vi "Apply Gate.vi"(8 "nramp":i32, 9 "Waveform in":dbl[](array[numeric])) -> (1 "Gated waveform":dbl[](array[numeric]))   [LabVIEW 2020]
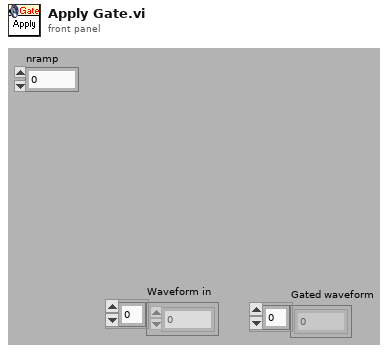
[diagram p1: front panel]
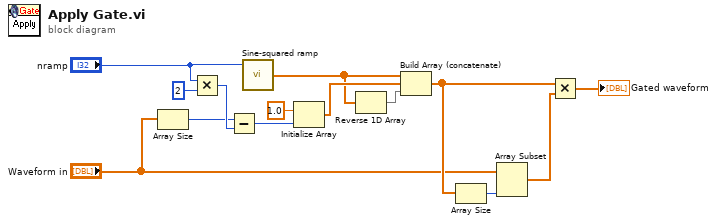
[diagram p0: block diagram]
diagram:
  n1 = Array Size(array="Waveform in") -> (size(s)=w2:i32)
  n2 = Multiply(x="nramp", y=2) -> (x*y=w13:i32)
  n3 = Subtract(x=w2, y=w13) -> (x-y=w12:i32)
  n4 = call "Sine-squared ramp.vi"("samples"="nramp") -> ("sine^2 Ramp"=w5:dbl[])  [unwired: 3 in, 1 out]
  n5 = Initialize Array(1.0 ("element"), w12) -> (w10:dbl[])
  n6 = Reverse 1D Array(array=w5) -> (reversed array=w9:dbl[])
  n7 = Build Array (concatenate)(w5, w10, w9) -> (w6:dbl[])
  n8 = Array Size(array=w6) -> (size(s)=w8:i32)
  n9 = Array Subset(array="Waveform in", length=w8) -> (w7:dbl[])  [unwired: 1 in]
  n10 = Multiply(x=w6, y=w7) -> (x*y=→"Gated waveform":dbl[])
